vi "MB Ethernet String to Modbus Data Unit.vi"(8 "error in (no error)":errorcluster, 11 "String":string) -> (0 "error out":errorcluster, 1 "Exception Code":u8 format="%.0x", 3 "Modbus Data Unit":T1={"Function Code"=1, "Data"=[]} {"Function Code" items=["Read Coils"=1, "Read Discrete Inputs"=2, "Read Holding Registers"=3, "Read Input Registers"=4, "Write Single Coil"=5, "Write Single Register"=6, "Read Exception Status"=7, "Write Multiple Coils"=15, "Write Multiple Registers"=16]; "Data" format="%.0x"})   [LabVIEW 2023, in "Voegtlin_NI_SMART_Modbus_Drivers.lvlib"]
uses:
  Voegtlin_NI_SMART_Modbus_Drivers.lvlib
  MB Modbus Data Unit.ctl
panel:
  # "VI Name: MB Ethernet String to Modbus Data Unit.vi\nPurpose: Formats the string received through Ethernet in a Modbus Data Unit.\nReentrant VI because its caller is also reentrant."
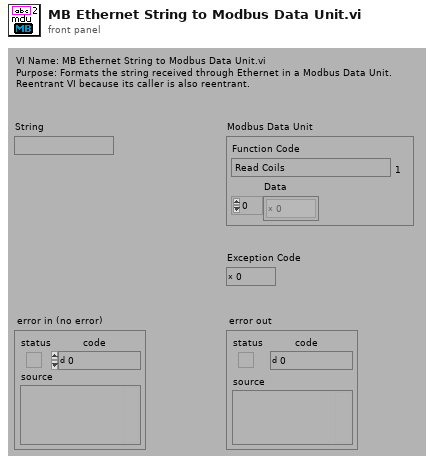
[diagram p1: front panel]
types:
  T1 = typedef "Voegtlin_NI_SMART_Modbus_Drivers.lvlib/MB Modbus Data Unit.ctl" = cluster{"Function Code":u8, "Data":u8[]}
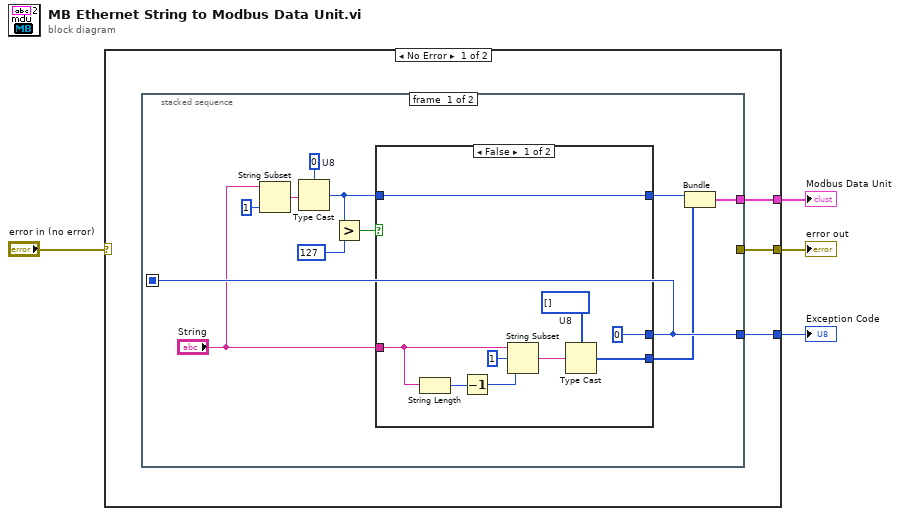
[diagram p0: block diagram]
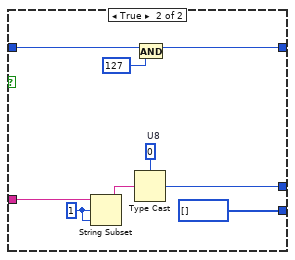
[diagram p2: hidden frame]
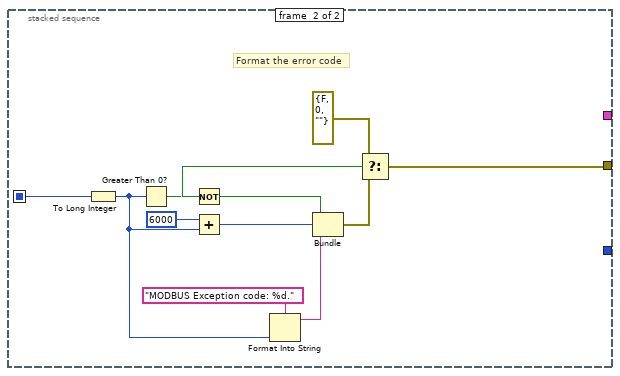
[diagram p3: hidden frame]
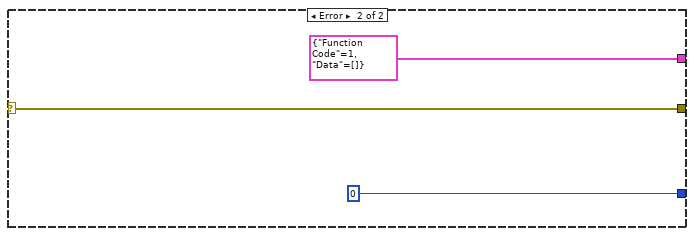
[diagram p4: hidden frame]
diagram:
  n1 = case shown="No Error" "error in (no error)" {
    selector: "error in (no error)" -> [_ w50]
    tunnel: [w7 u8 0 ("U8")] -> w4
    tunnel: [w6 w50] -> w2
    tunnel: [w5 T1 {"Function Code"=1, "Data"=[]} ("MODBUS Data Unit")] -> w1
    frame No Error {
      n2 = stacked-sequence {
        seq-local: [w18 _] -> [_ w41]
        tunnel: [w18 _] -> w7
        tunnel: [_ w40] -> w6
        tunnel: [w15 _] -> w5
        frame #0 {
          w13 = u8 0  # U8
          n3 = String Subset(string="String", length (rest)=1) -> (substring=w14:string)  [unwired: 1 out]
          n4 = Type Cast(type=w13, x=w14) -> (*(type *) &x=w10:u8)
          n5 = Greater?(x=w10, y=u8 127) -> (0:w11:bool)
          n6 = case shown="False" w11 {
            tunnel: "String" -> [w26 w31]
            tunnel: [w24 u8[] [] ("U8")] -> w17
            tunnel: [u8 0 w30] -> w18
            tunnel: w10 -> [w22 w35]
            tunnel: [w22 w34] -> w16
            frame False {
              w21 = u8[] []  # U8
              n7 = String Length(string=w26) -> (length=w19:i32)
              n8 = Decrement(x=w19) -> (x-1=w20:i32)
              n9 = String Subset(string=w26, offset (0)=1, length (rest)=w20) -> (substring=w25:string)
              n10 = Type Cast(type=w21, x=w25) -> (*(type *) &x=w24:u8[])
            }
            frame True {
              w33 = u8 0  # U8
              w28 = 1
              n11 = String Subset(string=w31, offset (0)=w28, length (rest)=w28) -> (substring=w32:string)
              n12 = Type Cast(type=w33, x=w32) -> (*(type *) &x=w30:u8)
              n13 = And(x=w35, y=u8 127) -> (x .and. y?=w34:u8)
            }
          }
          n14 = Bundle("U8"=w16, "U8"=w17) -> (w15:cluster{"U8":u8, "U8":u8[]})  [unwired: 1 out]
        }
        frame #1 {
          # "Format the error code"
          n15 = To Long Integer(number=w41) -> (32bit integer=w37:i32)
          n16 = Greater Than 0?(x=w37) -> (x > 0?=w44:bool)
          n17 = Not(x=w44) -> (.not. x?=w45:bool)
          n18 = Add(x=6000 ("New Error Code"), y=w37) -> (x+y=w39:i32)
          n19 = Format Into String(format string="MODBUS Exception code: %d.", w37) -> (resulting string=w43:string)  [unwired: 2 in, 1 out]
          n20 = Bundle(w44, w39, w43) -> (w46:errorcluster)  [unwired: 1 out]
          n21 = Select(t=errorcluster {"status"=FALSE, "code"=0, "source"=""} ("error out"), s=w45, f=w46) -> (s? t:f=w40:errorcluster)
        }
      }
    }
    frame Error {
    }
  }
  "error out" <- w2
  "Exception Code" <- w4
  "Modbus Data Unit" <- w1
